vi "Read jav pos.vi"(8 "error in (no error)":errorcluster, 11 "Constant Jerk Guidance in":refnum<class "Constant Jerk Guidance.lvclass">) -> (0 "error out":errorcluster, 2 "jav pos":dbl[](array[numeric])=[0.2, 0.2, 0.3], 3 "Constant Jerk Guidance out":refnum<class "Constant Jerk Guidance.lvclass">)   [LabVIEW 2014, in "Guidance Library.lvlib" / "Constant Jerk Guidance.lvclass"]
uses:
  Constant Jerk Guidance.lvclass
  Constant Jerk Guidance.lvclass/Constant Jerk Guidance.ctl
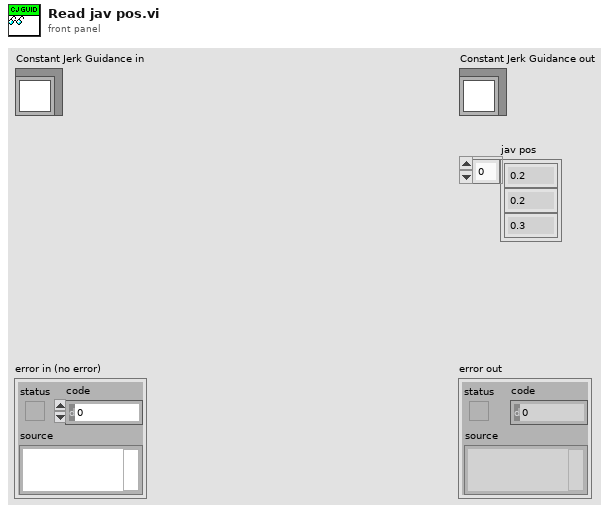
[diagram p1: front panel]
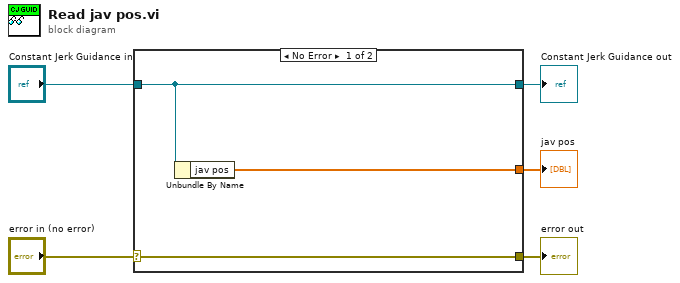
[diagram p0: block diagram]
diagram:
  n1 = case shown="No Error" "error in (no error)" {
    selector: "error in (no error)" -> [w8 w9]
    tunnel: [w8 w9] -> w4
    tunnel: [w7 w10] -> w2
    tunnel: "Constant Jerk Guidance in" -> [w7 w10]
    tunnel: [w6 _] -> w1
    frame No Error {
      n2 = Unbundle By Name(w7) -> ("jav pos"=w6:dbl[])
    }
    frame Error {
    }
  }
  "error out" <- w4
  "Constant Jerk Guidance out" <- w2
  "jav pos" <- w1
